vi "Pulse Counter.vi"(7 "Interval":T1(ring), 9 "B":bool, 11 "A":bool) -> (3 "Count":i32)   [LabVIEW 2014]
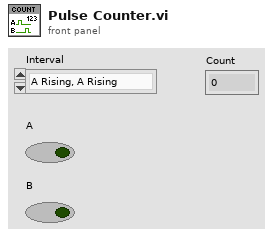
[diagram p1: front panel]
types:
  T1 = enum16{"A Rising, A Rising", "A Rising, A Falling", "A Falling, A Rising", "A Falling, A Falling", "A Rising, B Rising", "A Rising, B Falling", "A Falling, B Rising", "A Falling, B Falling"}
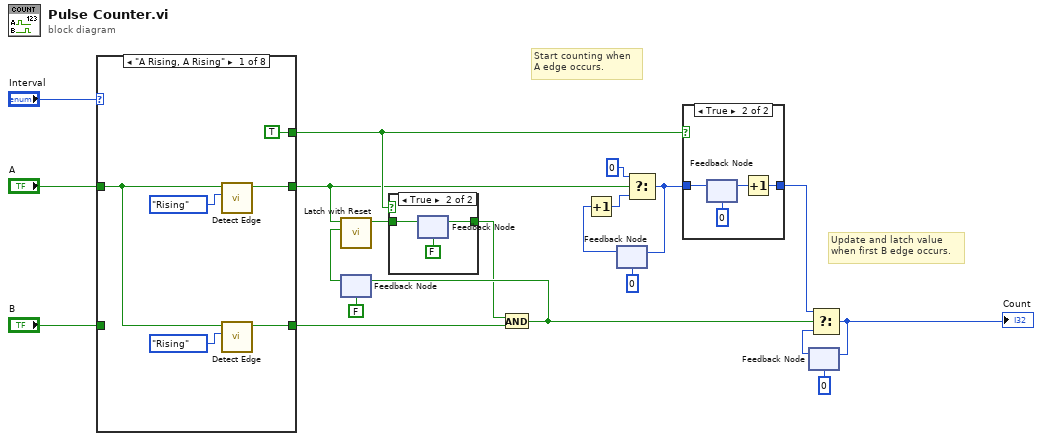
[diagram p0: block diagram]
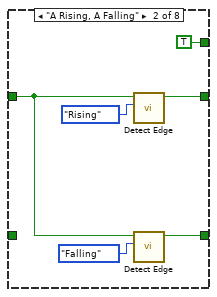
[diagram p4: hidden frame]
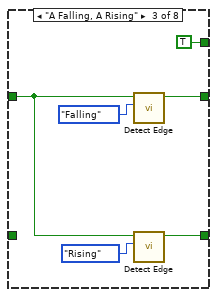
[diagram p5: hidden frame]
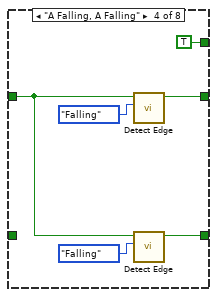
[diagram p6: hidden frame]
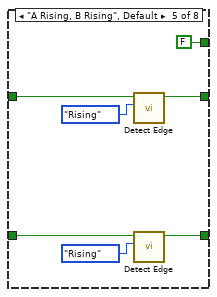
[diagram p7: hidden frame]
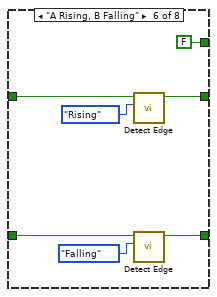
[diagram p8: hidden frame]
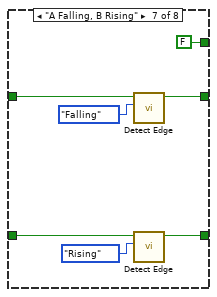
[diagram p9: hidden frame]
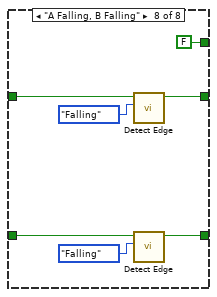
[diagram p10: hidden frame]
diagram:
  # "Update and latch value\nwhen first B edge occurs."
  # "Start counting when\nA edge occurs."
  n1 = case shown="\"A Rising, A Rising\"" "Interval" {
    tunnel: "A" -> [w24 w30 w36 w42 w50 w56 w63 w70]
    tunnel: "B" -> [_ _ _ _ w48 w55 w62 w69]
    tunnel: [w23 w29 w35 w41 w47 w54 w60 w68] -> w1
    tunnel: [w22 w28 w34 w40 w46 w53 w61 w67] -> w9
    tunnel: [TRUE TRUE TRUE TRUE FALSE FALSE FALSE FALSE] -> w4
    frame "A Rising, A Rising" {
      n2 = call "Detect Edge.vi"("Edge Type?"=enum16{"Rising", "Falling"}."Rising", "Signal In"=w24) -> ("Edge Detected?"=w23:bool)  [unwired: 9 in]
      n3 = call "Detect Edge.vi"("Edge Type?"=enum16{"Rising", "Falling"}."Rising", "Signal In"=w24) -> ("Edge Detected?"=w22:bool)  [unwired: 9 in]
    }
    frame "A Rising, A Falling" {
      n4 = call "Detect Edge.vi"("Edge Type?"=enum16{"Rising", "Falling"}."Rising", "Signal In"=w30) -> ("Edge Detected?"=w29:bool)  [unwired: 9 in]
      n5 = call "Detect Edge.vi"("Edge Type?"=enum16{"Rising", "Falling"}."Falling", "Signal In"=w30) -> ("Edge Detected?"=w28:bool)  [unwired: 9 in]
    }
    frame "A Falling, A Rising" {
      n6 = call "Detect Edge.vi"("Edge Type?"=enum16{"Rising", "Falling"}."Falling", "Signal In"=w36) -> ("Edge Detected?"=w35:bool)  [unwired: 9 in]
      n7 = call "Detect Edge.vi"("Edge Type?"=enum16{"Rising", "Falling"}."Rising", "Signal In"=w36) -> ("Edge Detected?"=w34:bool)  [unwired: 9 in]
    }
    frame "A Falling, A Falling" {
      n8 = call "Detect Edge.vi"("Edge Type?"=enum16{"Rising", "Falling"}."Falling", "Signal In"=w42) -> ("Edge Detected?"=w41:bool)  [unwired: 9 in]
      n9 = call "Detect Edge.vi"("Edge Type?"=enum16{"Rising", "Falling"}."Falling", "Signal In"=w42) -> ("Edge Detected?"=w40:bool)  [unwired: 9 in]
    }
    frame "A Rising, B Rising", Default {
      n10 = call "Detect Edge.vi"("Edge Type?"=enum16{"Rising", "Falling"}."Rising", "Signal In"=w50) -> ("Edge Detected?"=w47:bool)  [unwired: 9 in]
      n11 = call "Detect Edge.vi"("Edge Type?"=enum16{"Rising", "Falling"}."Rising", "Signal In"=w48) -> ("Edge Detected?"=w46:bool)  [unwired: 9 in]
    }
    frame "A Rising, B Falling" {
      n12 = call "Detect Edge.vi"("Edge Type?"=enum16{"Rising", "Falling"}."Rising", "Signal In"=w56) -> ("Edge Detected?"=w54:bool)  [unwired: 9 in]
      n13 = call "Detect Edge.vi"("Edge Type?"=enum16{"Rising", "Falling"}."Falling", "Signal In"=w55) -> ("Edge Detected?"=w53:bool)  [unwired: 9 in]
    }
    frame "A Falling, B Rising" {
      n14 = call "Detect Edge.vi"("Edge Type?"=enum16{"Rising", "Falling"}."Falling", "Signal In"=w63) -> ("Edge Detected?"=w60:bool)  [unwired: 9 in]
      n15 = call "Detect Edge.vi"("Edge Type?"=enum16{"Rising", "Falling"}."Rising", "Signal In"=w62) -> ("Edge Detected?"=w61:bool)  [unwired: 9 in]
    }
    frame "A Falling, B Falling" {
      n16 = call "Detect Edge.vi"("Edge Type?"=enum16{"Rising", "Falling"}."Falling", "Signal In"=w70) -> ("Edge Detected?"=w68:bool)  [unwired: 9 in]
      n17 = call "Detect Edge.vi"("Edge Type?"=enum16{"Rising", "Falling"}."Falling", "Signal In"=w69) -> ("Edge Detected?"=w67:bool)  [unwired: 9 in]
    }
  }
  n18 = feedback #1(FALSE ("Signal Out")) -> (w10:bool)
  n19 = call "Latch with Reset.vi"("Reset"=w10, "Signal In"=w1) -> ("Signal Out"=w6:bool)  [unwired: 9 in]
  n20 = case shown="True" w4 {
    tunnel: w6 -> [w73 w75]
    tunnel: [w73 w74] -> w5
    frame False {
    }
    frame True {
      n21 = feedback #2(FALSE ("Signal Out")) -> (w74:bool)
      n22 = feedback-in #2(w75) -> ()
    }
  }
  n23 = And(x=w5, y=w9) -> (x .and. y?=w8:bool)
  n24 = feedback-in #1(w8) -> ()
  n25 = feedback #3(0 ("Simulation Ticks")) -> (w11:i32)
  n26 = Increment(x=w11) -> (x+1=w15:i32)
  n27 = Select(t=0, s=w1, f=w15) -> (s? t:f=w3:i32)
  n28 = feedback-in #3(w3) -> ()
  n29 = case shown="True" w4 {
    tunnel: w3 -> [w77 w81]
    tunnel: [w77 w78] -> w2
    frame False {
    }
    frame True {
      n30 = feedback #4(0 ("Simulation Ticks")) -> (w80:i32)
      n31 = feedback-in #4(w81) -> ()
      n32 = Increment(x=w80) -> (x+1=w78:i32)
    }
  }
  n33 = feedback #5(0 ("Simulation Ticks")) -> (w13:i32)
  n34 = Select(t=w2, s=w8, f=w13) -> (s? t:f=w12:i32)
  "Count" <- w12
  n35 = feedback-in #5(w12) -> ()
